vi "CRYPlot XY Graph Preview.vi"(10 "sOption":string, 11 "Graph VI Ref":refnum<vi>) -> ()   [LabVIEW 2013]
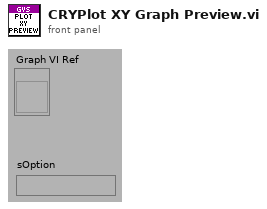
[diagram p1: front panel]
types:
  T1 = cluster{"Cursor.Cursor X":dbl, "YScale.Maximum":dbl}
  T2 = cluster{cluster{"Cursor.Cursor X":dbl, "YScale.Maximum":dbl}[]}
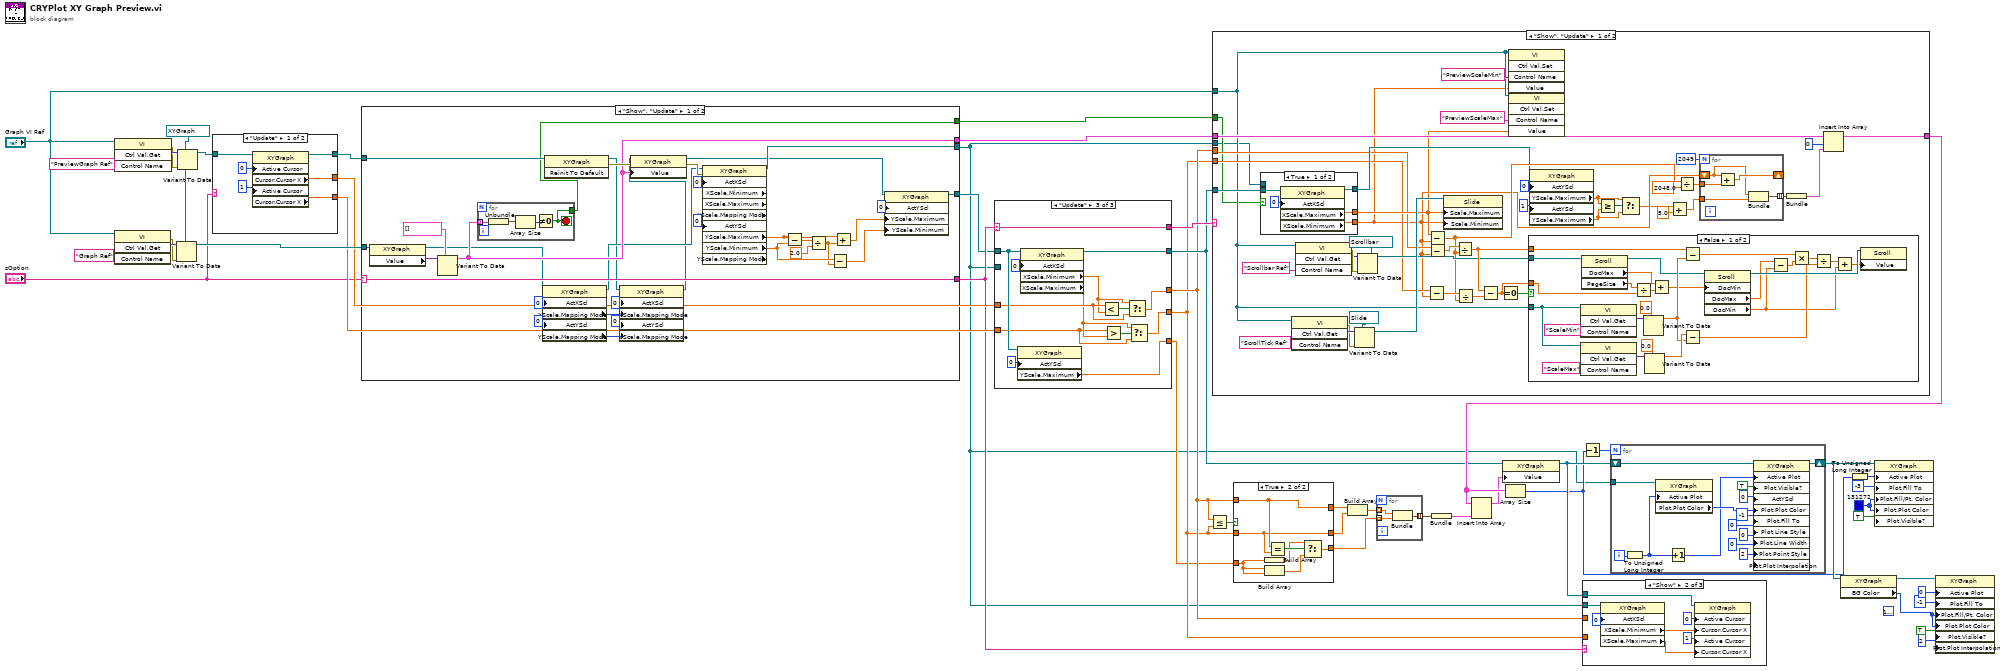
[diagram p0: block diagram]
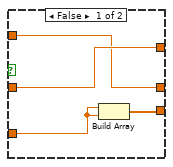
[diagram p2: hidden frame]
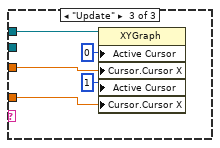
[diagram p5: hidden frame]
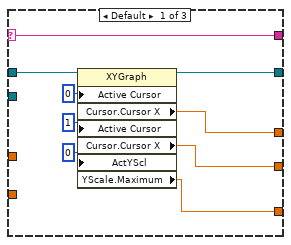
[diagram p6: hidden frame]
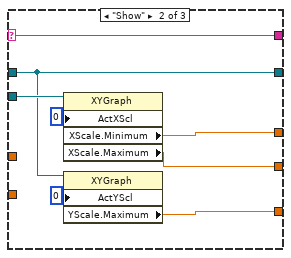
[diagram p7: hidden frame]
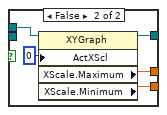
[diagram p8: hidden frame]
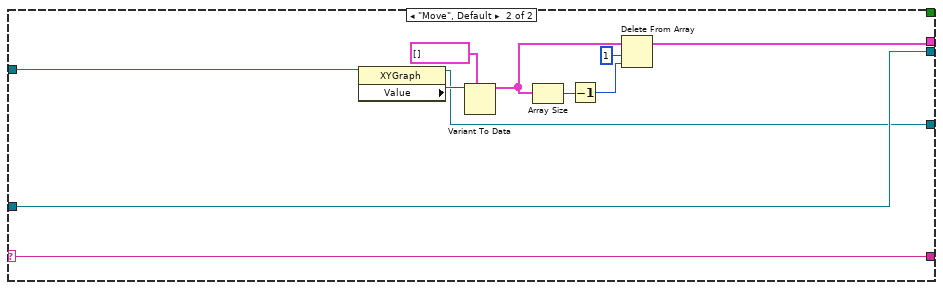
[diagram p11: hidden frame]
diagram:
  (unwired) u32 16777226
  w18 = u32 131272
  w40 = refnum<vi> refnum ("Legend Ref")
  n1 = invoke class="VI" method="Ctrl Val.Get"(reference="Graph VI Ref", "Control Name"="Graph Ref") -> (error out=w42:errorcluster, "Get Control Value Variant"=w43:variant)  [unwired: 2 in, 2 out]
  n2 = invoke class="VI" method="Ctrl Val.Get"(reference="Graph VI Ref", "Control Name"="PreviewGraph Ref") -> (error out=w46:errorcluster, "Get Control Value Variant"=w47:variant)  [unwired: 2 in, 2 out]
  n3 = Variant To Data(error in=w42, type=w40, Variant=w43) -> (data=w41:refnum<vi>)  [unwired: 1 out]
  n4 = Variant To Data(error in=w46, type=w40, Variant=w47) -> (data=w30:refnum<vi>)  [unwired: 1 out]
  n5 = case shown="\"Update\"" "sOption" {
    tunnel: [w53 w54] -> w29
    tunnel: [w52 _] -> w27
    tunnel: [w51 _] -> w28
    tunnel: w30 -> [w48 w54]
    frame "Update" {
      n6 = property on="Property Node" class="XYGraph"(reference=w48, "Active Cursor"=u32 0, "Active Cursor"=u32 1) -> (reference out=w53:refnum<vi>, "Cursor.Cursor X"=w51:dbl, "Cursor.Cursor X"=w52:dbl)  [unwired: 1 in, 1 out]
    }
    frame "Show", Default {
    }
  }
  n7 = case shown="\"Show\", \"Update\"" "sOption" {
    selector: "sOption" -> [w78 w92]
    tunnel: w29 -> [w86 w94]
    tunnel: w41 -> [w81 w101]
    tunnel: [w83 w93] -> w24
    tunnel: [w77 w101] -> w2
    tunnel: [w66 w95] -> w39
    tunnel: [w78 w92] -> w26
    tunnel: [w65 _] -> w3
    frame "Show", "Update" {
      n8 = property class="XYGraph"(reference=w81) -> (reference out=w58:refnum<vi>, "Value"=w82:variant)  [unwired: 1 in, 1 out]
      n9 = Variant To Data(type=cluster{cluster{"x":dbl, "z":dbl}[]}[] [], Variant=w82) -> (data=w66:cluster{cluster{"x":dbl, "z":dbl}[]}[])  [unwired: 1 in, 1 out]
      n10 = for {
        tunnel: w66 -> [w90] mode=indexing
        tunnel: [w87] -> w65
        stop <- w87 stop-if-true
        n11 = Unbundle(w90) -> (w89:cluster{"x":dbl, "z":dbl}[])
        n12 = Array Size(array=w89) -> (size(s)=w88:i32)
        n13 = Not Equal To 0?(x=w88) -> (x != 0?=w87:bool)
      }
      n14 = property on="Property Node" class="XYGraph"(reference=w58, "ActXScl"=0 ("Active Y Scale"), "ActYScl"=0 ("Active Y Scale")) -> (reference out=w57:refnum<vi>, "XScale.Mapping Mode"=w63:u8, "YScale.Mapping Mode"=w64:u8)  [unwired: 1 in, 1 out]
      n15 = invoke class="XYGraph" method="Reinit To Default"(reference=w86) -> (reference out=w56:refnum<vi>, error out=w79:errorcluster)  [unwired: 2 in, 1 out]
      n16 = property on="Property Node" class="XYGraph"(reference=w56, "ActXScl"=0 ("Active Y Scale"), "XScale.Mapping Mode"=w63, "ActYScl"=0 ("Active Y Scale"), "YScale.Mapping Mode"=w64) -> (reference out=w55:refnum<vi>)  [unwired: 1 in, 1 out]
      n17 = property class="XYGraph"(reference=w55, error in=w79, "Value"=w66) -> (reference out=w69:refnum<vi>, error out=w80:errorcluster)
      n18 = property on="Property Node" class="XYGraph" props=["ActXScl", "XScale", "Minimum", "XScale", "Maximum", "XScale", "Mapping Mode", "ActYScl", "YScale", "Maximum", "YScale", "Minimum", "YScale", "Mapping Mode"](reference=w57, error in=w80, "ActXScl"=0 ("Active Y Scale"), "ActYScl"=0 ("Active Y Scale")) -> (reference out=w77:refnum<vi>, "YScale.Maximum"=w73:dbl, "YScale.Minimum"=w72:dbl)  [unwired: 5 out]
      n19 = Subtract(x=w73, y=w72) -> (x-y=w76:dbl)
      n20 = Divide(x=w76, y=2.0) -> (x/y=w70:dbl)
      n21 = Subtract(x=w72, y=w70) -> (x-y=w71:dbl)
      n22 = Add(x=w73, y=w70) -> (x+y=w74:dbl)
      n23 = property on="Property Node" class="XYGraph"(reference=w69, "ActYScl"=0 ("Active Y Scale"), "YScale.Maximum"=w74, "YScale.Minimum"=w71) -> (reference out=w83:refnum<vi>)  [unwired: 1 in, 1 out]
    }
    frame "Move", Default {
      n24 = property class="XYGraph"(reference=w94) -> (reference out=w93:refnum<vi>, "Value"=w100:variant)  [unwired: 1 in, 1 out]
      n25 = Variant To Data(type=cluster{cluster{"x":dbl, "z":dbl}[]}[] [], Variant=w100) -> (data=w98:cluster{cluster{"x":dbl, "z":dbl}[]}[])  [unwired: 1 in, 1 out]
      n26 = Array Size(array=w98) -> (size(s)=w97:i32)
      n27 = Decrement(x=w97) -> (x-1=w96:i32)
      n28 = Delete From Array(array=w98, length=1, index=w96) -> (array with subset deleted=w95:cluster{cluster{"x":dbl, "z":dbl}[]}[])  [unwired: 1 out]
    }
  }
  n29 = case shown="\"Update\"" w26 {
    selector: w26 -> [w102 w111 w119]
    tunnel: [w110 w113 w130] -> w12
    tunnel: [w109 w112 w120] -> w23
    tunnel: [w107 w115 w121] -> w21
    tunnel: [w106 w116 w126] -> w22
    tunnel: w24 -> [w103 w112 w129]
    tunnel: w2 -> [_ w117 _]
    tunnel: w28 -> [_ _ w127]
    tunnel: w27 -> [_ _ w122]
    tunnel: [w102 w111 w119] -> w25
    frame Default {
      n30 = property on="Property Node" class="XYGraph"(reference=w103, "Active Cursor"=u32 0, "Active Cursor"=u32 1, "ActYScl"=0 ("Active Y Scale")) -> (reference out=w109:refnum<vi>, "Cursor.Cursor X"=w106:dbl, "Cursor.Cursor X"=w107:dbl, "YScale.Maximum"=w110:dbl)  [unwired: 1 in, 1 out]
    }
    frame "Show" {
      n31 = property on="Property Node" class="XYGraph"(reference=w117, "ActXScl"=0 ("Active Y Scale")) -> ("XScale.Minimum"=w116:dbl, "XScale.Maximum"=w115:dbl)  [unwired: 1 in, 2 out]
      n32 = property on="Property Node" class="XYGraph"(reference=w112, "ActYScl"=0 ("Active Y Scale")) -> ("YScale.Maximum"=w113:dbl)  [unwired: 1 in, 2 out]
    }
    frame "Update" {
      n33 = property on="Property Node" class="XYGraph"(reference=w129, "ActYScl"=0 ("Active Y Scale")) -> ("YScale.Maximum"=w130:dbl)  [unwired: 1 in, 2 out]
      n34 = property on="Property Node" class="XYGraph"(reference=w129, "ActXScl"=0 ("Active Y Scale")) -> (reference out=w120:refnum<vi>, "XScale.Minimum"=w125:dbl, "XScale.Maximum"=w123:dbl)  [unwired: 1 in, 1 out]
      n35 = Less?(x=w127, y=w125) -> (x < y?=w128:bool)
      n36 = Greater?(x=w122, y=w123) -> (0:w124:bool)
      n37 = Select(t=w125, s=w128, f=w127) -> (s? t:f=w126:dbl)
      n38 = Select(t=w123, s=w124, f=w122) -> (s? t:f=w121:dbl)
    }
  }
  n39 = Less Or Equal?(x=w22, y=w21) -> (x <= y?=w15:bool)
  n40 = case shown="\"Show\", \"Update\"" w25 {
    tunnel: "Graph VI Ref" -> [w148 _]
    tunnel: w23 -> [w162 _]
    tunnel: w39 -> [w160 w218]
    tunnel: [w153 w218] -> w38
    tunnel: w22 -> [w150 _]
    tunnel: w21 -> [w149 _]
    tunnel: w3 -> [w134 _]
    tunnel: w2 -> [w133 _]
    frame "Show", "Update" {
      n41 = case shown="True" w134 {
        tunnel: w162 -> [w181 _]
        tunnel: [w180 w186] -> w157
        tunnel: [w179 w185] -> w154
        tunnel: [w177 w183] -> w144
        tunnel: w133 -> [_ w182]
        frame True {
          n42 = property on="Property Node" class="XYGraph"(reference=w181, "ActXScl"=0 ("Active X Scale")) -> (reference out=w180:refnum<vi>, "XScale.Maximum"=w179:dbl, "XScale.Minimum"=w177:dbl)  [unwired: 1 in, 1 out]
        }
        frame False {
          n43 = property on="Property Node" class="XYGraph"(reference=w182, "ActXScl"=0 ("Active X Scale")) -> (reference out=w186:refnum<vi>, "XScale.Maximum"=w185:dbl, "XScale.Minimum"=w183:dbl)  [unwired: 1 in, 1 out]
        }
      }
      n44 = invoke class="VI" method="Ctrl Val.Get"(reference=w148, "Control Name"="ScrollTick Ref") -> (error out=w169:errorcluster, "Get Control Value Variant"=w170:variant)  [unwired: 2 in, 2 out]
      n45 = invoke class="VI" method="Ctrl Val.Get"(reference=w148, "Control Name"="Scrollbar Ref") -> (error out=w164:errorcluster, "Get Control Value Variant"=w163:variant)  [unwired: 2 in, 2 out]
      n46 = Variant To Data(error in=w169, type=refnum<vi> refnum ("Legend Ref"), Variant=w170) -> (data=w172:refnum<vi>)  [unwired: 1 out]
      n47 = Variant To Data(error in=w164, type=refnum<vi> refnum ("Legend Ref"), Variant=w163) -> (data=w166:refnum<vi>)  [unwired: 1 out]
      n48 = Subtract(x=w149, y=w144) -> (x-y=w175:dbl)
      n49 = Subtract(x=w154, y=w144) -> (x-y=w158:dbl)
      n50 = Subtract(x=w150, y=w144) -> (x-y=w173:dbl)
      n51 = property on="Property Node" class="Slide"(reference=w172, "Scale.Maximum"=w154, "Scale.Minimum"=w144) -> ()  [unwired: 1 in, 2 out]
      n52 = Divide(x=w173, y=w158) -> (x/y=w174:dbl)
      n53 = Divide(x=w175, y=w158) -> (x/y=w176:dbl)
      n54 = Subtract(x=w174, y=w176) -> (x-y=w146:dbl)
      n55 = Equal To 0?(x=w146) -> (x = 0?=w147:bool)
      n56 = invoke class="VI" method="Ctrl Val.Set"(reference=w148, "Control Name"="PreviewScaleMin", "Value"=w144) -> ()  [unwired: 2 in, 5 out]
      n57 = invoke class="VI" method="Ctrl Val.Set"(reference=w148, "Control Name"="PreviewScaleMax", "Value"=w154) -> ()  [unwired: 2 in, 5 out]
      n58 = case shown="False" w147 {
        tunnel: w174 -> [w217 _]
        tunnel: w166 -> [w216 _]
        tunnel: w148 -> [w193 _]
        tunnel: w146 -> [w192 _]
        frame False {
          n59 = invoke class="VI" method="Ctrl Val.Get"(reference=w193, "Control Name"="ScaleMin") -> ("Get Control Value Variant"=w210:variant)  [unwired: 2 in, 3 out]
          n60 = invoke class="VI" method="Ctrl Val.Get"(reference=w193, "Control Name"="ScaleMax") -> ("Get Control Value Variant"=w213:variant)  [unwired: 2 in, 3 out]
          n61 = property on="Property Node" class="Scroll"(reference=w216) -> (reference out=w206:refnum<vi>, "DocMax"=w203:dbl, "PageSize"=w196:dbl)  [unwired: 1 in, 1 out]
          n62 = Divide(x=w196, y=w192) -> (x/y=w205:dbl)
          n63 = Variant To Data(type=0.0 ("X Scale.Range:Maximum"), Variant=w210) -> (data=w214:dbl)  [unwired: 1 in, 1 out]
          n64 = Variant To Data(type=0.0 ("X Scale.Range:Maximum"), Variant=w213) -> (data=w215:dbl)  [unwired: 1 in, 1 out]
          n65 = Add(x=w203, y=w205) -> (x+y=w204:dbl)
          n66 = Subtract(x=w217, y=w214) -> (x-y=w202:dbl)
          n67 = Subtract(x=w215, y=w214) -> (x-y=w199:dbl)
          n68 = property on="Property Node" class="Scroll"(reference=w206, "DocMin"=w204) -> (reference out=w207:refnum<vi>, "DocMax"=w194:dbl, "DocMin"=w195:dbl)  [unwired: 1 in, 1 out]
          n69 = Subtract(x=w194, y=w195) -> (x-y=w201:dbl)
          n70 = Multiply(x=w202, y=w201) -> (x*y=w200:dbl)
          n71 = Divide(x=w200, y=w199) -> (x/y=w198:dbl)
          n72 = Add(x=w198, y=w195) -> (x+y=w197:dbl)
          n73 = property on="Property Node" class="Scroll"(reference=w207, "Value"=w197) -> ()  [unwired: 1 in, 2 out]
        }
        frame True {
        }
      }
      n74 = property on="Property Node" class="XYGraph"(reference=w157, "ActYScl"=0 ("Active Y Scale"), "ActYScl"=1 ("Active Y Scale")) -> ("YScale.Maximum"=w137:dbl, "YScale.Maximum"=w136:dbl)  [unwired: 1 in, 2 out]
      n75 = Greater Or Equal?(x=w137, y=w136) -> (x >= y?=w138:bool)
      n76 = Select(t=w137, s=w138, f=w136) -> (s? t:f=w135:dbl)
      n77 = Add(x=w135, y=5.0) -> (x+y=w142:dbl)
      n78 = Divide(x=w158, y=2048.0) -> (x/y=w145:dbl)
      n79 = for {
        N: 2049 ("dimension size") -> [_]
        tunnel: w145 -> [w191]
        shift-right: [w190] -> _
        shift-left: w144 -> [w189]
        tunnel: w142 -> [w188]
        tunnel: [w187] -> w141 mode=indexing
        n80 = Add(x=w189, y=w191) -> (x+y=w190:dbl)
        n81 = Bundle("XScale.Minimum"=w189, w188) -> (w187:cluster{"XScale.Minimum":dbl, dbl})  [unwired: 1 in]
      }
      n82 = Bundle(w141) -> (w140:cluster{cluster{"XScale.Minimum":dbl, dbl}[]})  [unwired: 1 in]
      n83 = Insert Into Array(array=w160, index=0, new element=w140) -> (w153:cluster{cluster{"x":dbl, "z":dbl}[]}[])
    }
    frame Default {
    }
  }
  n84 = case shown="True" w15 {
    tunnel: [w222 w229] -> w9
    tunnel: w22 -> [w221 w229]
    tunnel: [w221 w228] -> w8
    tunnel: w21 -> [w222 w228]
    tunnel: w12 -> [w220 w224]
    tunnel: [w219 w225] -> w10
    frame False {
      n85 = Build Array(w220, w220) -> (w219:dbl[])
    }
    frame True {
      n86 = Build Array(w224) -> (w223:dbl[])
      n87 = Build Array(w224, w224) -> (w226:dbl[])
      n88 = Equal?(x=w229, y=w228) -> (x = y?=w227:bool)
      n89 = Select(t=w223, s=w227, f=w226) -> (s? t:f=w225:dbl[])
    }
  }
  n90 = Build Array(w9, w8) -> (w7:dbl[])
  n91 = for {
    tunnel: [w232] -> w11 mode=indexing
    tunnel: w10 -> [w231] mode=indexing
    tunnel: w7 -> [w230] mode=indexing
    n92 = Bundle("Cursor.Cursor X"=w230, "YScale.Maximum"=w231) -> (w232:T1)  [unwired: 1 in]
  }
  n93 = Bundle(w11) -> (w6:T2)  [unwired: 1 in]
  n94 = Insert Into Array(array=w38, new element=w6) -> (w16:cluster{cluster{"x":dbl, "z":dbl}[]}[])  [unwired: 1 in]
  n95 = property class="XYGraph"(reference=w23, "Value"=w16) -> (reference out=w31:refnum<vi>)  [unwired: 1 in, 1 out]
  n96 = Array Size(array=w38) -> (size(s)=w14:i32)
  n97 = Decrement(x=w14) -> (x-1=w13:i32)
  n98 = case shown="\"Show\"" w26 {
    tunnel: w31 -> [_ w234 w242]
    tunnel: w2 -> [_ w233 _]
    tunnel: w22 -> [_ _ w241]
    tunnel: w21 -> [_ _ w240]
    frame Default {
    }
    frame "Show" {
      n99 = property on="Property Node" class="XYGraph"(reference=w233, "ActXScl"=0 ("Active Y Scale")) -> ("XScale.Minimum"=w238:dbl, "XScale.Maximum"=w239:dbl)  [unwired: 1 in, 2 out]
      n100 = property on="Property Node" class="XYGraph"(reference=w234, "Active Cursor"=u32 0, "Cursor.Cursor X"=w238, "Active Cursor"=u32 1, "Cursor.Cursor X"=w239) -> ()  [unwired: 1 in, 2 out]
    }
    frame "Update" {
      n101 = property on="Property Node" class="XYGraph"(reference=w242, "Active Cursor"=u32 0, "Cursor.Cursor X"=w241, "Active Cursor"=u32 1, "Cursor.Cursor X"=w240) -> ()  [unwired: 1 in, 2 out]
    }
  }
  n102 = for {
    N: w13 -> [_]
    shift-right: [w249] -> w32
    shift-left: w31 -> [w250]
    tunnel: w2 -> [w247]
    i -> [w251]
    n103 = To Unsigned Long Integer(number=w251) -> (unsigned 32bit integer=w246:u32)
    n104 = property class="XYGraph"(reference=w247, "Active Plot"=w246) -> ("Plot.Plot Color"=w248:u32)  [unwired: 1 in, 2 out]
    n105 = Increment(x=w246) -> (x+1=w245:u32)
    n106 = property class="XYGraph"(reference=w250, "Active Plot"=w245, "Plot.Visible?"=TRUE ("Plot.Visible"), "ActYScl"=0 ("Active Y Scale"), "Plot.Plot Color"=w248, "Plot.Fill To"=i16 -1, "Plot.Line Style"=u8 0, "Plot.Line Width"=u8 0, "Plot.Point Style"=u8 0, "Plot.Plot Interpolation"=u8 2) -> (reference out=w249:refnum<vi>)  [unwired: 1 in, 1 out]
  }
  n107 = property on="Property Node" class="XYGraph"(reference=w32) -> (reference out=w33:refnum<vi>, "BG Color"=w1:u32)  [unwired: 1 in, 1 out]
  n108 = To Unsigned Long Integer(number=w14) -> (unsigned 32bit integer=w20:u32)
  n109 = property on="Property Node" class="XYGraph"(reference=w32, "Active Plot"=w20, "Plot.Fill To"=i16 -3, "Plot.Fill/Pt. Color"=w18, "Plot.Plot Color"=w18, "Plot.Visible?"=TRUE ("Plot.Visible")) -> ()  [unwired: 1 in, 2 out]
  n110 = property on="Property Node" class="XYGraph"(reference=w33, "Active Plot"=u32 0, "Plot.Fill To"=i16 -1, "Plot.Fill/Pt. Color"=w1, "Plot.Plot Color"=w1, "Plot.Visible?"=TRUE ("Plot.Visible"), "Plot.Plot Interpolation"=u8 2) -> ()  [unwired: 1 in, 2 out]
